vi "Terminate.vi"(8 "error in (no error)":errorcluster, 10 "Message in":refnum<class "TerminateMessage.lvclass">, 11 "BMC in":refnum<class "BMC.lvclass">) -> (0 "error out":errorcluster, 3 "BMC out":refnum<class "BMC.lvclass">)   [LabVIEW 2012, in "BMC.lvclass"]
doc: "This member function is called when the statemachine in the run.vi receives an 'terminate' command. It closes the RabbitMQ connection. \n\nOverride this member function in your derived class to release all previously acquired resources (but don't forget to call the parent method). If your component has subcomponents, they count as resources, and you have to release them by calling their own terminate functions."
uses:
  BMC.lvclass
  <vilib>/Distrio/Murmex/TerminateMessage/TerminateMessage.lvclass
  <vilib>/Distrio/Murmex/Murmex/Murmex.lvclass
panel:
  # "This method is called when the TERMINATE\ntrigger is sent. \n\nOverride this method when your component needs to\nrespond to this trigger. \n\nCall parent for proper implementation"
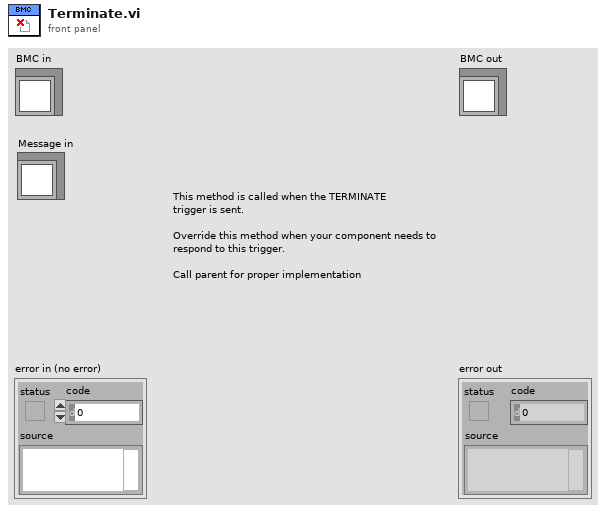
[diagram p1: front panel]
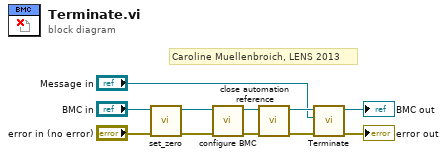
[diagram p0: block diagram]
diagram:
  # "Caroline Muellenbroich, LENS 2013"
  n1 = call-dynamic "set_zero.vi"("error in (no error)"="error in (no error)", "BMC in"="BMC in") -> ("error out"=w5:errorcluster, "BMC out"=w6:refnum<class "BMC.lvclass">)  [unwired: 8 in]
  n2 = call-dynamic "configure BMC.vi"("error in (no error)"=w5, "BMC in"=w6) -> ("error out"=w4:errorcluster, "BMC out"=w3:refnum<class "BMC.lvclass">)  [unwired: 8 in]
  n3 = call-dynamic "close automation reference.vi"("error in (no error)"=w4, "BMC in"=w3) -> ("error out"=w9:errorcluster, "BMC out"=w8:refnum<class "BMC.lvclass">)  [unwired: 8 in]
  n4 = call-parent "Terminate.vi"("error in (no error)"=w9, "Message in"="Message in", "Murmex in"=w8) -> ("error out"=→"error out":errorcluster, "Murmex out"=→"BMC out":refnum<class "BMC.lvclass">)  [unwired: 7 in]
